vi "Get ini file info block from text string.vi"(8 "error in (no error)":errorcluster, 10 "Section key":string, 11 "String":string) -> (0 "error out":errorcluster, 2 "Found section info":bool, 3 "Info block":string)   [LabVIEW 2013]
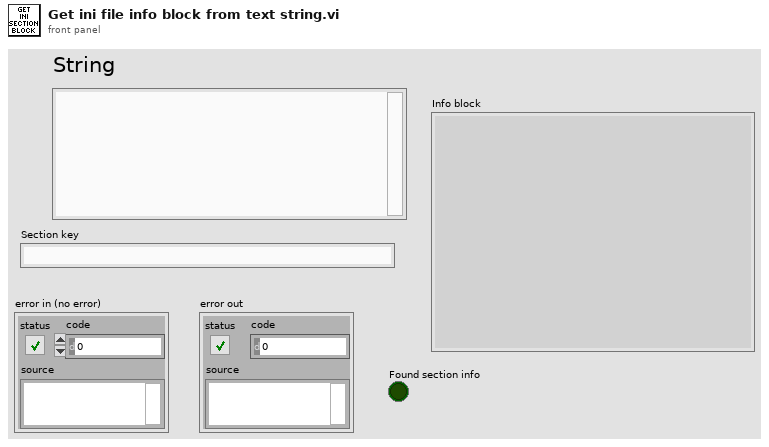
[diagram p1: front panel]
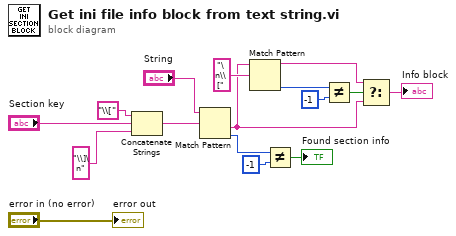
[diagram p0: block diagram]
diagram:
  n1 = Concatenate Strings("\\[" ("string"), "Section key", "\\]\n" ("string")) -> (w15:string)
  n2 = Match Pattern(string="String", regular expression=w15) -> (after substring=w5:string, offset past match=w2:i32)  [unwired: 1 in, 2 out]
  n3 = Match Pattern(string=w5, regular expression="\n\\[") -> (before substring=w6:string, offset past match=w11:i32)  [unwired: 1 in, 2 out]
  n4 = Not Equal?(x=w2, y=-1) -> (x != y?=→"Found section info":bool)
  n5 = Not Equal?(x=w11, y=-1) -> (x != y?=w7:bool)
  n6 = Select(t=w6, s=w7, f=w5) -> (s? t:f=→"Info block":string)
  "error out" <- "error in (no error)"
